vi "Get Is BlackLevel Supported.vi"(8 "error in (no error)":errorcluster, 11 "TLCamera reference in":refnum<k24>) -> (0 "error out":errorcluster, 2 "Is BlackLevel Supported?":bool, 3 "TLCamera reference out":refnum<k24>)   [LabVIEW 2020]
uses:
  C:/GEECS/Developers Version/source/Device Drivers/Point Grey Camera/Library_X86/Thorlabs.TSI.TLCameraInterfaces.dll
  Point Grey Camera/Library_X86/Thorlabs.TSI.TLCameraInterfaces.dll
  C:/GEECS/Developers Version/source/Device Drivers/Point Grey Camera/Library_X86/Thorlabs.TSI.CoreInterfaces.dll
  Point Grey Camera/Library_X86/Thorlabs.TSI.CoreInterfaces.dll
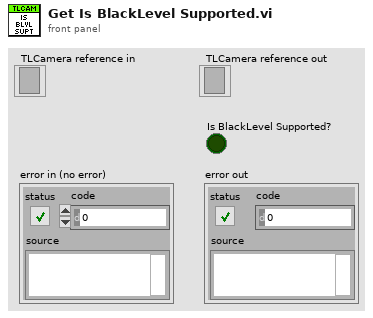
[diagram p1: front panel]
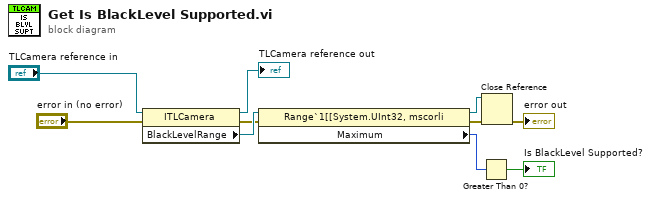
[diagram p0: block diagram]
diagram:
  n1 = property class="ITLCamera"(reference="TLCamera reference in", error in="error in (no error)") -> (reference out=→"TLCamera reference out":refnum<k24>, error out=w8:errorcluster, "BlackLevelRange"=w9:refnum<k24>)
  n2 = property class="Range`1[[System.UInt32, mscorli"(reference=w9, error in=w8) -> (reference out=w3:refnum<k24>, error out=w2:errorcluster, "Maximum"=w5:u32)
  n3 = Greater Than 0?(x=w5) -> (x > 0?=→"Is BlackLevel Supported?":bool)
  n4 = Close Reference(reference=w3, error in (no error)=w2) -> (error out=→"error out":errorcluster)
